vi "VRMS_DC_Filter_compute.vi"(0 "CH0 Data":dbl[](array[numeric]), 1 "CH0 Shift V":dbl, 2 "CH0 multiplier":dbl, 3 "CH1 multiplier":dbl, 5 "CH1 Data":dbl[](array[numeric]), 9 "DC filter ON/OFF":bool, 11 "Number Of Samples":dbl, 13 "CH1 Shift V":dbl) -> (4 "CH1 Vave":dbl, 6 "CH2 Vave":dbl, 10 "CH1RMS":dbl, 12 "CH0 Y array":dbl[](array[numeric]), 14 "CH1 Y array":dbl[](array[numeric]), 15 "CH2RMS":dbl)   [LabVIEW 2012]
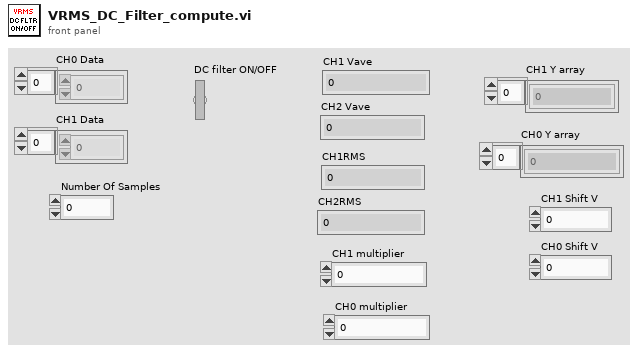
[diagram p1: front panel]
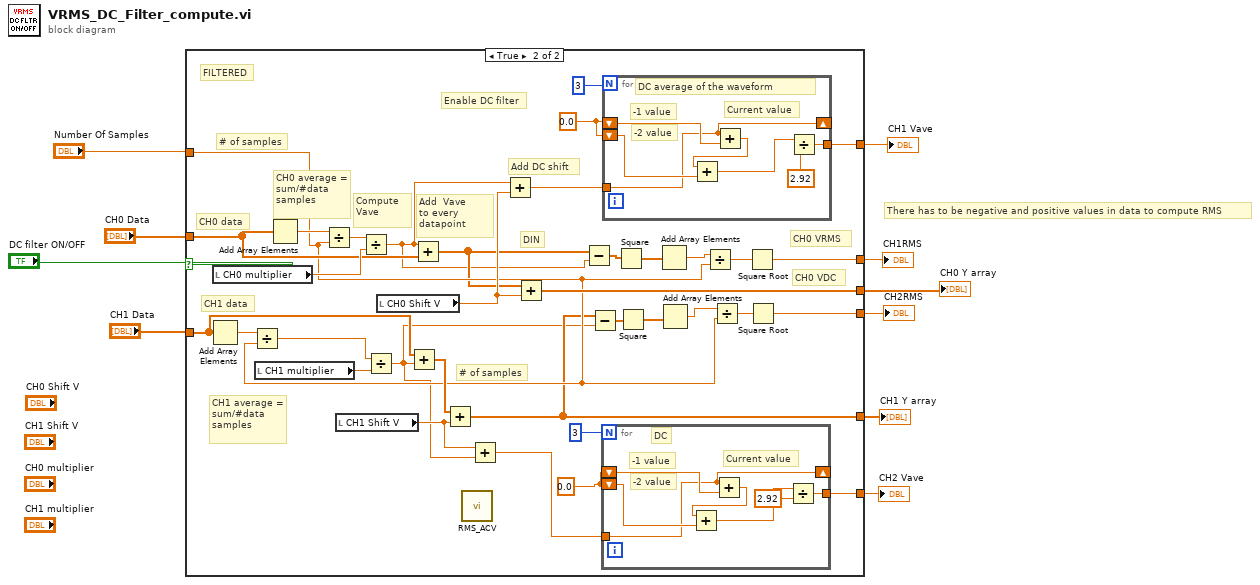
[diagram p0: block diagram]
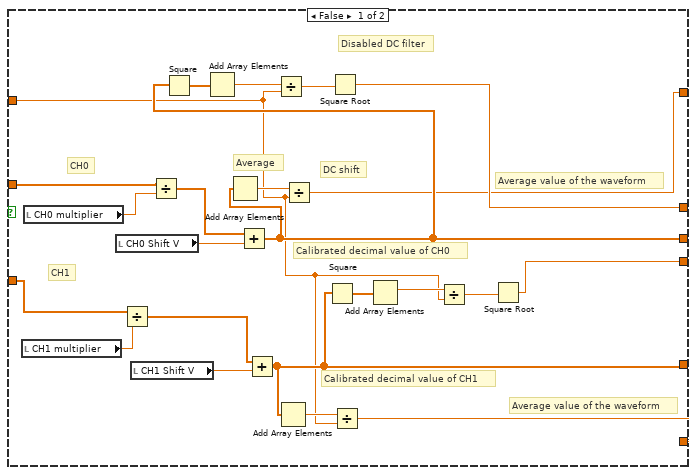
[diagram p2: hidden frame]
diagram:
  # "There has to be negative and positive values in data to compute RMS"
  n1 = case shown="True" "DC filter ON/OFF" {
    tunnel: "CH0 Data" -> [w13 w53]
    tunnel: "CH1 Data" -> [w33 w52]
    tunnel: [w19 w41] -> w2
    tunnel: [w20 w49] -> w1
    tunnel: [w15 w56] -> w3
    tunnel: [w16 w60] -> w6
    tunnel: "Number Of Samples" -> [w17 w44]
    tunnel: [w27 w36] -> w5
    tunnel: [w21 w35] -> w4
    frame False {
      # "CH1"
      # "CH0"
      # "Average value of the waveform"
      # "Average value of the waveform"
      # "Disabled DC filter"
      # "Calibrated decimal value of CH1"
      # "Calibrated decimal value of CH0"
      # "DC shift"
      # "Average"
      n2 = local read "CH1 multiplier"() -> (w32:dbl)
      n3 = local read "CH0 multiplier"() -> (w11:dbl)
      n4 = local read "CH0 Shift V"() -> (w29:dbl)
      n5 = Divide(x=w33, y=w32) -> (x/y=w22:dbl[])
      n6 = local read "CH1 Shift V"() -> (w31:dbl)
      n7 = Divide(x=w13, y=w11) -> (x/y=w12:dbl[])
      n8 = Add(x=w12, y=w29) -> (x+y=w20:dbl[])
      n9 = Square(x=w20) -> (x^2=w28:dbl[])
      n10 = Add Array Elements(numeric array=w28) -> (sum=w14:dbl)
      n11 = Add Array Elements(numeric array=w20) -> (sum=w30:dbl)
      n12 = Add(x=w22, y=w31) -> (x+y=w19:dbl[])
      n13 = Divide(x=w14, y=w17) -> (x/y=w26:dbl)
      n14 = Add Array Elements(numeric array=w19) -> (sum=w18:dbl)
      n15 = Divide(x=w30, y=w17) -> (x/y=w16:dbl)
      n16 = Square(x=w19) -> (x^2=w25:dbl[])
      n17 = Square Root(x=w26) -> (sqrt(x)=w27:dbl)
      n18 = Divide(x=w18, y=w17) -> (x/y=w15:dbl)
      n19 = Add Array Elements(numeric array=w25) -> (sum=w23:dbl)
      n20 = Divide(x=w23, y=w17) -> (x/y=w24:dbl)
      n21 = Square Root(x=w24) -> (sqrt(x)=w21:dbl)
    }
    frame True {
      w57 = 0.0
      w62 = 0.0
      # "DIN"
      # "Enable DC filter"
      # "FILTERED"
      # "CH1 average = sum/#data samples"
      # "CH0 VRMS"
      # "CH0 VDC"
      # "Add DC shift"
      # "Compute Vave"
      # "# of samples"
      # "# of samples"
      # "CH1 data"
      # "CH0 data"
      # "Add  Vave\nto every datapoint"
      # "CH0 average = sum/#data samples"
      n22 = Add Array Elements(numeric array=w52) -> (sum=w67:dbl)
      n23 = local read "CH0 multiplier"() -> (w64:dbl)
      n24 = Divide(x=w67, y=w44) -> (x/y=w66:dbl)
      n25 = local read "CH1 multiplier"() -> (w63:dbl)
      n26 = Add Array Elements(numeric array=w53) -> (sum=w68:dbl)
      n27 = Divide(x=w68, y=w44) -> (x/y=w42:dbl)
      n28 = local read "CH1 Shift V"() -> (w55:dbl)
      n29 = Divide(x=w42, y=w64) -> (x/y=w39:dbl)
      n30 = Divide(x=w66, y=w63) -> (x/y=w40:dbl)
      n31 = local read "CH0 Shift V"() -> (w59:dbl)
      n32 = Add(x=w52, y=w40) -> (x+y=w65:dbl[])
      n33 = Add(x=w39, y=w53) -> (x+y=w43:dbl[])
      n34 = Add(x=w65, y=w55) -> (x+y=w41:dbl[])
      n35 = call "RMS_ACV.vi"() -> ()  [unwired: 11 in, 1 out]
      n36 = Add(x=w55, y=w40) -> (x+y=w54:dbl)
      n37 = Add(x=w39, y=w59) -> (x+y=w58:dbl)
      n38 = Add(x=w43, y=w59) -> (x+y=w49:dbl[])
      n39 = Subtract(x=w43, y=w39) -> (x-y=w37:dbl[])
      n40 = Subtract(x=w41, y=w40) -> (x-y=w38:dbl[])
      n41 = for {
        N: 3 -> [_]
        shift-right: [w69] -> _
        shift-left: w57 -> [w75]
        shift-left: w57 -> [w72]
        tunnel: [w70] -> w56
        tunnel: w54 -> [w69]
        # "DC"
        # "-2 value"
        # "-1 value"
        # "Current value"
        n42 = Add(x=w69, y=w75) -> (x+y=w73:dbl)
        n43 = Add(x=w73, y=w72) -> (x+y=w71:dbl)
        n44 = Divide(x=w71, y=2.92) -> (x/y=w70:dbl)
      }
      n45 = for {
        N: 3 -> [_]
        shift-right: [w76] -> _
        shift-left: w62 -> [w82]
        shift-left: w62 -> [w79]
        tunnel: [w77] -> w60
        tunnel: w58 -> [w76]
        # "DC average of the waveform"
        # "-2 value"
        # "-1 value"
        # "Current value"
        n46 = Add(x=w76, y=w82) -> (x+y=w80:dbl)
        n47 = Add(x=w80, y=w79) -> (x+y=w78:dbl)
        n48 = Divide(x=w78, y=2.92) -> (x/y=w77:dbl)
      }
      n49 = Square(x=w37) -> (x^2=w48:dbl[])
      n50 = Square(x=w38) -> (x^2=w45:dbl[])
      n51 = Add Array Elements(numeric array=w48) -> (sum=w50:dbl)
      n52 = Add Array Elements(numeric array=w45) -> (sum=w46:dbl)
      n53 = Divide(x=w50, y=w44) -> (x/y=w51:dbl)
      n54 = Divide(x=w46, y=w44) -> (x/y=w47:dbl)
      n55 = Square Root(x=w51) -> (sqrt(x)=w36:dbl)
      n56 = Square Root(x=w47) -> (sqrt(x)=w35:dbl)
    }
  }
  "CH1 Vave" <- w6
  "CH2 Vave" <- w3
  "CH1RMS" <- w5
  "CH2RMS" <- w4
  "CH1 Y array" <- w2
  "CH0 Y array" <- w1
